vi "SendCommand.vi"(8 "error":errorcluster, 10 "write buffer (don't include >\\r\\n)":string, 11 "VISA resource name":refnum<visa-resource-name>) -> (0 "error out":errorcluster, 2 "Response":string, 3 "VISA resource name out":refnum<visa-resource-name>)   [LabVIEW 2023, in "BigSkyControl.lvlib"]
uses:
  BigSkyControl.lvlib
panel:
  out "Read return count":u32
  in  "byte count":u32=1024
  out "Write return count":u32
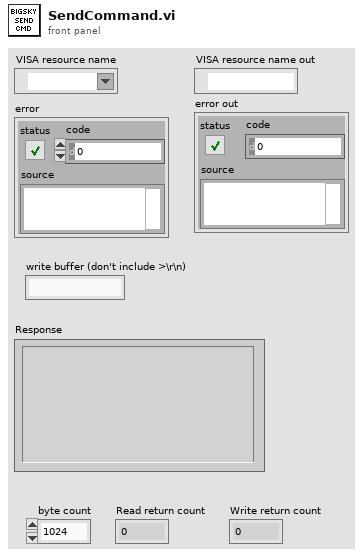
[diagram p1: front panel]
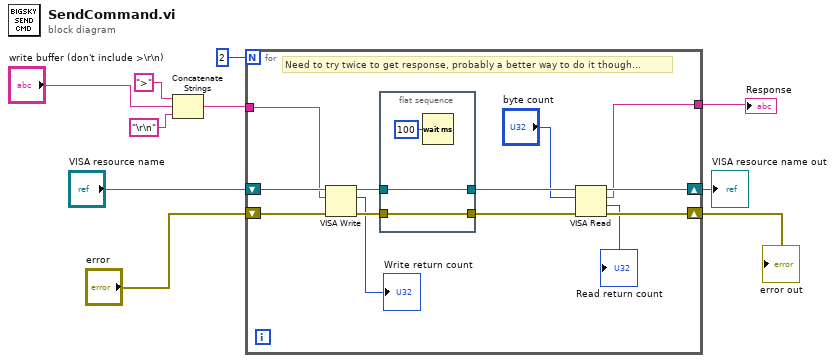
[diagram p0: block diagram]
diagram:
  n1 = Concatenate Strings(">" ("string"), "write buffer (don't include >\\r\\n)", "\r\n" ("write buffer")) -> (w2:string)
  n2 = for {
    N: 2 -> [_]
    shift-right: [w22] -> w7
    shift-left: "VISA resource name" -> [w21]
    shift-right: [w23] -> w6
    shift-left: "error" -> [w20]
    tunnel: [w12] -> w5
    tunnel: w2 -> [w11]
    # "Need to try twice to get response, probably a better way to do it though..."
    n3 = VISA Write(VISA resource name=w21, write buffer=w11, error in (no error)=w20) -> (VISA resource name out=w18:refnum<visa-resource-name>, return count=→"Write return count":u32, error out=w19:errorcluster)
    n4 = flat-sequence {
      tunnel: w19 -> [w26]
      tunnel: [w26] -> w16
      tunnel: w18 -> [w25]
      tunnel: [w25] -> w17
      frame #0 {
        n5 = Wait (ms)(milliseconds to wait=u32 100) -> ()  [unwired: 1 out]
      }
    }
    n6 = VISA Read(VISA resource name=w17, byte count="byte count", error in (no error)=w16) -> (VISA resource name out=w22:refnum<visa-resource-name>, read buffer=w12:string, return count=→"Read return count":u32, error out=w23:errorcluster)
  }
  "Response" <- w5
  "VISA resource name out" <- w7
  "error out" <- w6
